vi "Impedance to Capacitance.vi"(7 "Sweep Frequency Start":dbl, 8 "error in (no error)":errorcluster, 11 "Impedance":cdb[](array[numeric])) -> (0 "error out":errorcluster, 3 "Capacitance":dbl[](array[numeric]))   [LabVIEW 2013]
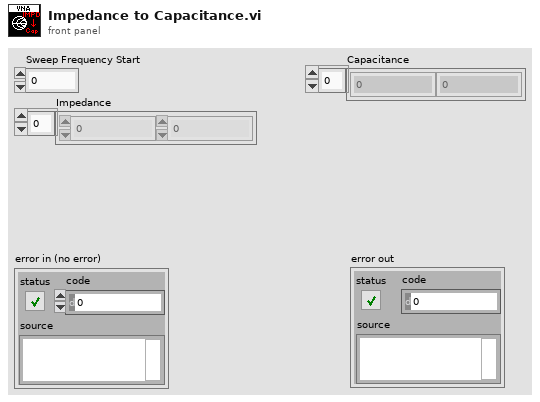
[diagram p1: front panel]
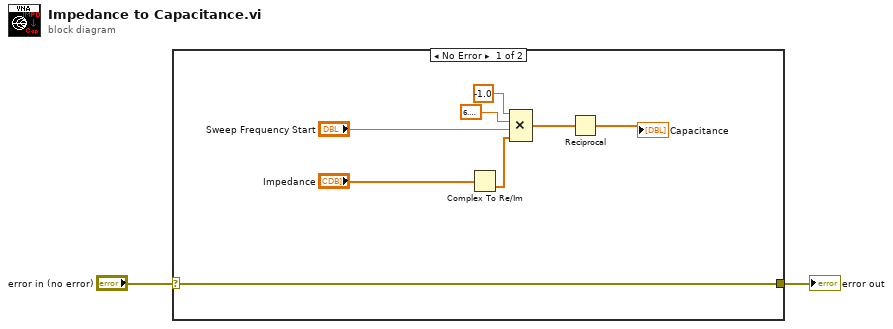
[diagram p0: block diagram]
diagram:
  n1 = case shown="No Error" "error in (no error)" {
    selector: "error in (no error)" -> [w7 w11]
    tunnel: [w7 w11] -> w2
    frame No Error {
      n2 = Complex To Re/Im(x + iy="Impedance") -> (y=w9:dbl[])  [unwired: 1 out]
      n3 = Compound Arithmetic op=MULTIPLY(-1.0, 6.283185307179586, "Sweep Frequency Start", w9) -> (w4:dbl[])
      n4 = Reciprocal(x=w4) -> (1/x=→"Capacitance":dbl[])
    }
    frame Error {
    }
  }
  "error out" <- w2
